vi "Handle Messages.vi"(8 "error in (no error)":errorcluster, 9 "Message Data":variant, 10 "Message":string, 11 "Worker In":refnum<class "Worker.lvclass">) -> (0 "error out":errorcluster, 3 "Worker Out":refnum<class "Worker.lvclass">)   [LabVIEW 2020, in "Worker.lvclass"]
uses:
  Worker.lvclass
  Person/Person.lvclass
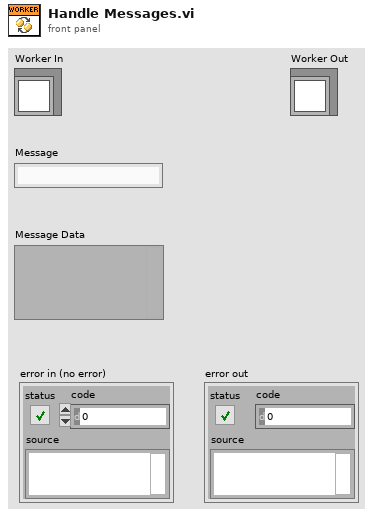
[diagram p1: front panel]
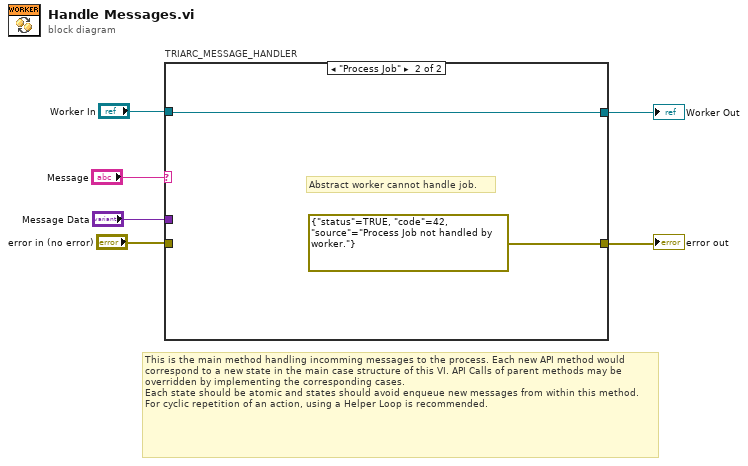
[diagram p0: block diagram]
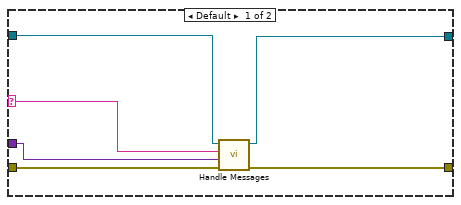
[diagram p2: hidden frame]
diagram:
  # "This is the main method handling incomming messages to the process. Each new API method would correspond to a new state in the main case structure of this VI. API Calls of parent methods may be overridden by implementing the corresponding cases.\nEach state should be atomic and states should avoid enqueue new messages from within this method. For cyclic repetition of an action, using a Helper Loop is recommended."
  n1 = case "TRIARC_MESSAGE_HANDLER" shown="\"Process Job\"" "Message" {
    selector: "Message" -> [w10 _]
    tunnel: "error in (no error)" -> [w9 _]
    tunnel: "Worker In" -> [w12 w14]
    tunnel: "Message Data" -> [w11 _]
    tunnel: [w8 errorcluster {"status"=TRUE, "code"=42, "source"="Process Job not handled by worker."} ("error out")] -> w2
    tunnel: [w7 w14] -> w1
    frame Default {
      n2 = call-parent "Handle Messages.vi"("error in (no error)"=w9, "Message Data"=w11, "Message"=w10, "Person In"=w12) -> ("error out"=w8:errorcluster, "Person Out"=w7:refnum<class "Worker.lvclass">)  [unwired: 6 in]
    }
    frame "Process Job" {
      # "Abstract worker cannot handle job."
    }
  }
  "error out" <- w2
  "Worker Out" <- w1
